vi "camera.vi"() -> ()   [LabVIEW 2021]
uses:
  <vilib>/userDefined/High Color/IMAQdx.ctl
  <vilib>/vision/driver/NI_Vision_Acquisition_Software.lvlib
panel:
  in  "확인 버튼":bool
  out "Image Out":T1(plugin-control)
  in  "정지":bool
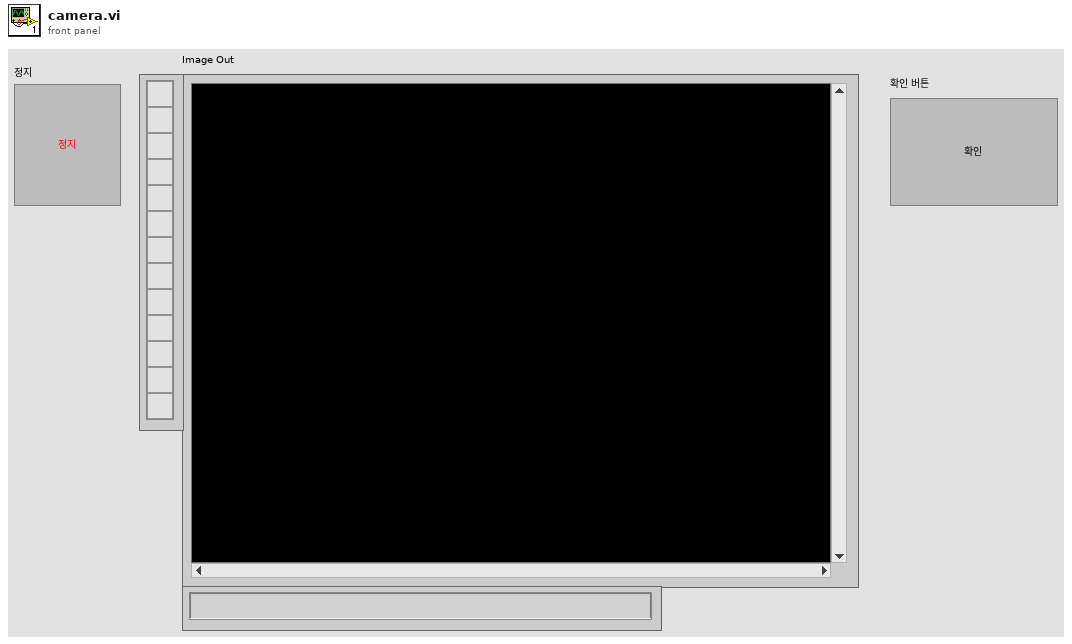
[diagram p1: front panel]
types:
  T1 = typedef "IMAQ Image.ctl" = refnum<image>
  T2 = typedef "Image Type" = u32
  T3 = typedef "IMAQdx.ctl" = refnum<k21>
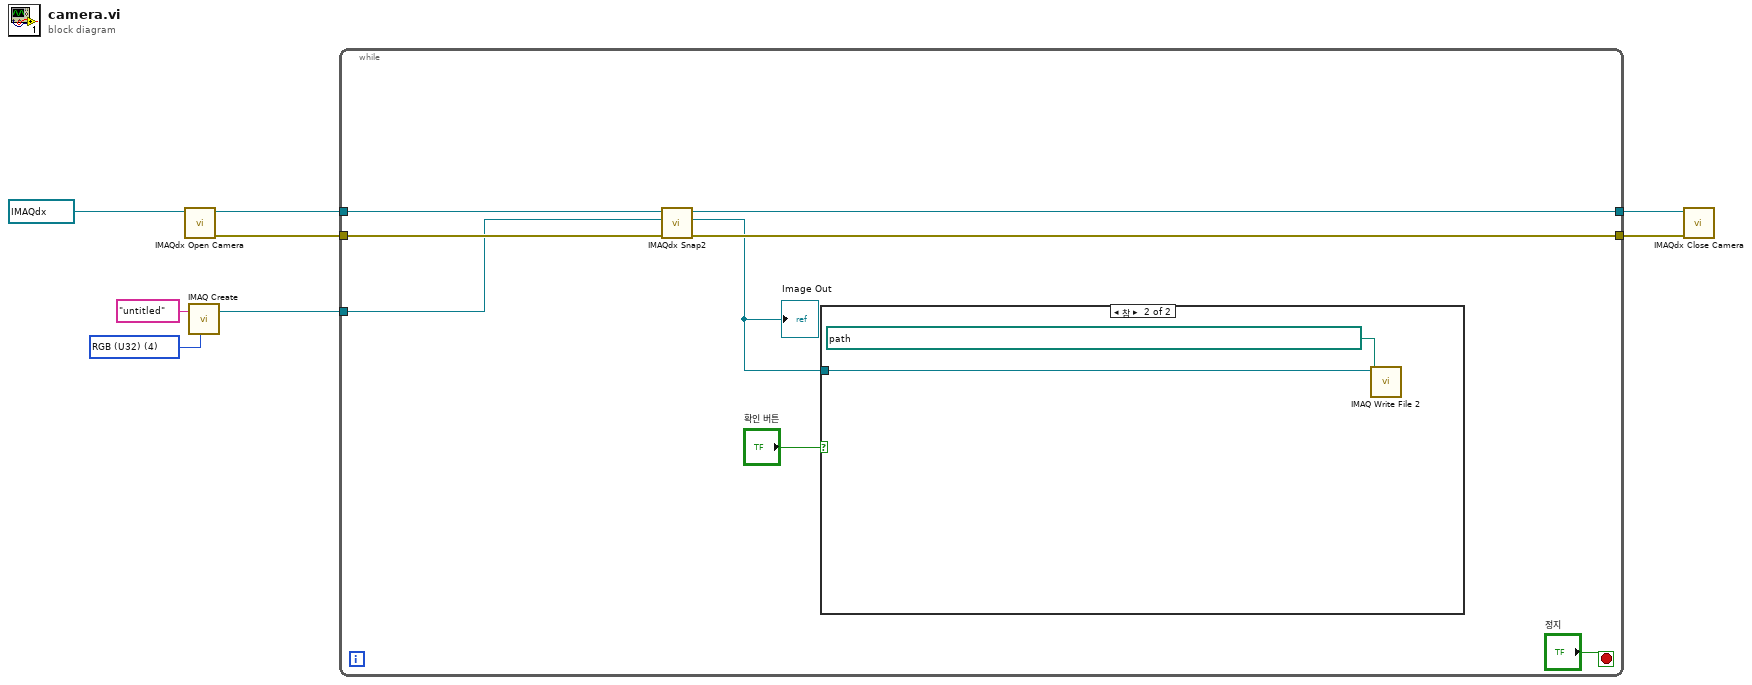
[diagram p0: block diagram]
diagram:
  w2 = T2 4 items=["Grayscale (U8)", "Grayscale (I16)", "Grayscale (SGL)", "Complex (CSG)", "RGB (U32)", "HSL (U32)", "RGB (U64)", "Grayscale (U16)"] ("Image Type")
  n1 = call <vilib>:"IMAQdx Open Camera.vi"("Session In"=T3 "cam0") -> ("error out"=w6:errorcluster, "Session Out"=w7:T3)  [unwired: 9 in]
  n2 = call "IMAQ Create"("Image Name"="untitled", "Image Type"=w2) -> ("New Image"=w1:T1)  [unwired: 3 in, 1 out]
  n3 = while {
    tunnel: w7 -> [w15]
    tunnel: w6 -> [w14]
    tunnel: [w13] -> w5
    tunnel: [w12] -> w4
    tunnel: w1 -> [w11]
    stop <- "정지" stop-if-true
    n4 = call <vilib>:"IMAQdx Snap2.vi"("error in"=w14, "Image In"=w11, "Session In"=w15) -> ("error out"=w12:errorcluster, "Image Out"=w9:T1, "Session Out"=w13:T3)  [unwired: 6 in]
    "Image Out" <- w9
    n5 = case shown="참" "확인 버튼" {
      tunnel: w9 -> [_ w18]
      frame False {
      }
      frame True {
        n6 = call-poly "IMAQ Write File 2"("File Path"=path "C:/Users/user/OneDrive/바탕 화면/Color_Dataset/Test/Test/Yellow0.jpg", "Image"=w18) -> ()  [unwired: 8 in, 2 out]
      }
    }
  }
  n7 = call <vilib>:"IMAQdx Close Camera.vi"("error in"=w4, "Session In"=w5) -> ()  [unwired: 9 in, 1 out]
